vi "Read results lookup table.vi"(8 "error in (no error)":errorcluster, 11 "Controller in":refnum<class "Controller.lvclass">) -> (0 "error out":errorcluster, 2 "results lookup table (function.timestamp -> results object)":variant, 3 "Controller out":refnum<class "Controller.lvclass">)   [LabVIEW 2016, in "Controller Actor.lvlib" / "Controller.lvclass"]
uses:
  <userlib>/Common Components/Controller/Controller.lvclass
  <userlib>/Common Components/Controller/Controller.lvclass/Controller.ctl
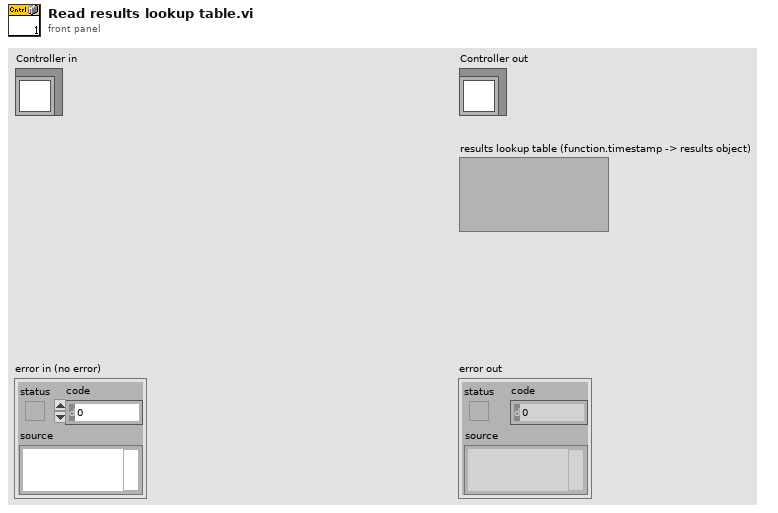
[diagram p1: front panel]
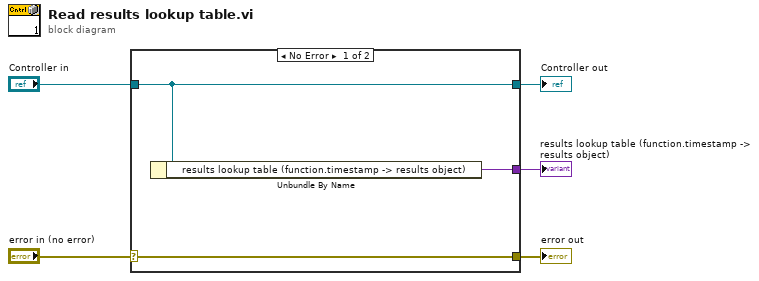
[diagram p0: block diagram]
diagram:
  n1 = case shown="No Error" "error in (no error)" {
    selector: "error in (no error)" -> [w8 w9]
    tunnel: [w8 w9] -> w4
    tunnel: [w7 w10] -> w2
    tunnel: "Controller in" -> [w7 w10]
    tunnel: [w6 _] -> w1
    frame No Error {
      n2 = Unbundle By Name(w7) -> ("results lookup table (function.timestamp -> results object)"=w6:variant)
    }
    frame Error {
    }
  }
  "error out" <- w4
  "Controller out" <- w2
  "results lookup table (function.timestamp -> results object)" <- w1
